vi "Vehicle Parameters (SubVI).vi"(9 "Nozzle eccentricity x/y [m] in":dbl[](array[numeric]), 10 "Nozzle misalignment yaw/pitch [º] in":dbl[](array[numeric]), 11 "dl [º]":dbl) -> (2 "Vehicle Parameters":T1)   [LabVIEW 2017]
panel:
  out "Nozzle misalignment yaw/pitch [º] out":dbl[](array[numeric])
  out "Nozzle eccentricity x/y [m] out":dbl[](array[numeric])
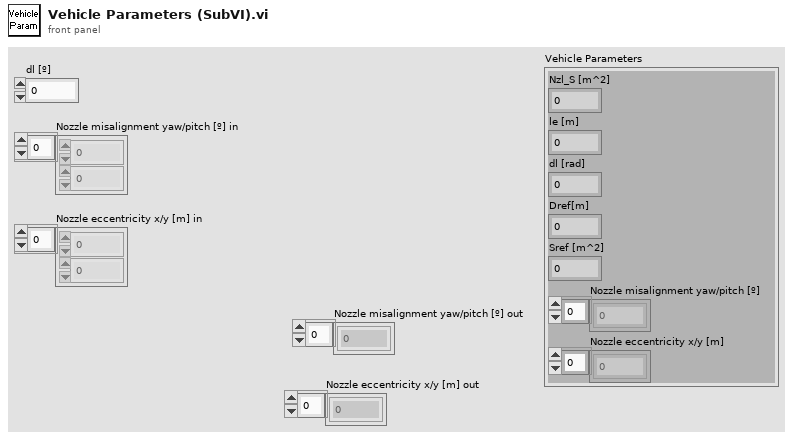
[diagram p1: front panel]
types:
  T1 = cluster{"Nzl_S [m^2]":dbl, "le [m]":dbl, "dl [rad]":dbl, "Dref[m]":dbl, "Sref [m^2]":dbl, "Nozzle misalignment yaw/pitch [º]":dbl[], "Nozzle eccentricity x/y [m]":dbl[]}
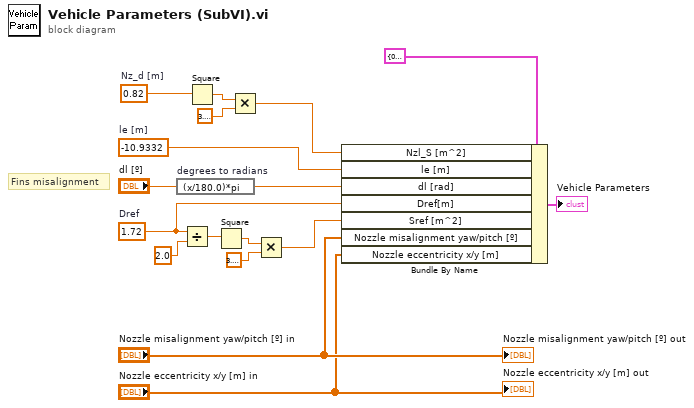
[diagram p0: block diagram]
diagram:
  w15 = 1.72  # Dref
  w8 = 0.82  # Nz_d [m]
  w13 = -10.9332  # le [m]
  # "Fins misalignment"
  n1 = expression code="(x/180.0)*pi" "degrees to radians"("dl [º]") -> (w14:dbl)
  n2 = Divide(x=w15, y=2.0) -> (x/y=w4:dbl)
  n3 = Square(x=w8) -> (x^2=w10:dbl)
  n4 = Square(x=w4) -> (x^2=w5:dbl)
  n5 = Multiply(x=w10, y=3.141592653589793) -> (x*y=w12:dbl)
  n6 = Multiply(x=w5, y=3.141592653589793) -> (x*y=w16:dbl)
  n7 = Bundle By Name(cluster=T1 {"Nzl_S [m^2]"=0.0, "le [m]"=-10.9332, "dl [rad]"=0.0, "Dref[m]"=1.72, "Sref [m^2]"=0.0, "Nozzle misalignment yaw/pitch [º]"=[], "Nozzle eccentricity x/y [m]"=[]} ("output cluster 2"), "Nzl_S [m^2]"=w12, "le [m]"=w13, "dl [rad]"=w14, "Dref[m]"=w15, "Sref [m^2]"=w16, "Nozzle misalignment yaw/pitch [º]"="Nozzle misalignment yaw/pitch [º] in", "Nozzle eccentricity x/y [m]"="Nozzle eccentricity x/y [m] in") -> (→"Vehicle Parameters":T1)
  "Nozzle eccentricity x/y [m] out" <- "Nozzle eccentricity x/y [m] in"
  "Nozzle misalignment yaw/pitch [º] out" <- "Nozzle misalignment yaw/pitch [º] in"
